vi "GetDAQOutputs.vi"(8 "error in (no error)":errorcluster, 11 "Device.Simulation in":refnum<class "Device.Simulation.lvclass">) -> (0 "error out":errorcluster, 2 "DAQ Outputs":T1, 3 "Device.Simulation out":refnum<class "Device.Simulation.lvclass">)   [LabVIEW 2019, in "Device.Simulation.lvlib" / "Device.Simulation.lvclass"]
uses:
  Device.Simulation.lvclass
  state--cluster.ctl
  Device.Simulation.lvclass/Device.Simulation.ctl
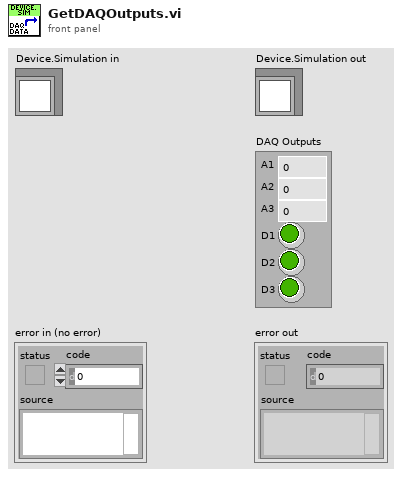
[diagram p1: front panel]
types:
  T1 = typedef "Device.Simulation.lvlib/Device.Simulation.lvclass/state--cluster.ctl" = cluster{"A1":dbl, "A2":dbl, "A3":dbl, "D1":bool, "D2":bool, "D3":bool}
  T2 = typedef "Device.Simulation.lvlib/Device.Simulation.lvclass/privateData--reference.ctl" = refnum<data-value>
  T3 = typedef "Device.Simulation.lvlib/Device.Simulation.lvclass/privateData--cluster.ctl" = cluster{"config":T4, "state":T1}
  T4 = typedef "Device.Simulation.lvlib/Device.Simulation.lvclass/config--cluster.ctl" = cluster{"Name":string, "Time to Connect (ms)":u32, "Time to Check Connection (ms)":u32, "Time to Disconnect (ms)":u32, "Time to Read State (ms)":u32}
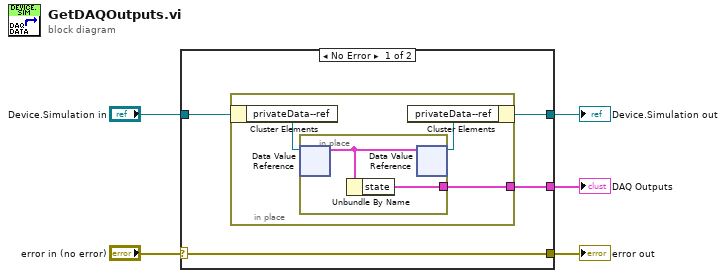
[diagram p0: block diagram]
diagram:
  n1 = case shown="No Error" "error in (no error)" {
    selector: "error in (no error)" -> [w9 w16]
    tunnel: [w9 w16] -> w4
    tunnel: [w7 w15] -> w2
    tunnel: "Device.Simulation in" -> [w8 w15]
    tunnel: [w6 _] -> w1
    frame No Error {
      n2 = in-place {
        in-place-border: [w12] -> w6
        n3 = in-place-cluster #1(w8) -> ("privateData--ref"=w11:T2)
        n4 = in-place {
          in-place-border: [w14] -> w12
          n5 = in-place-dvr #2(w11) -> (w13:T3)  [unwired: 1 out]
          n6 = Unbundle By Name(w13) -> ("state"=w14:T1)
          n7 = in-place-dvr #2(w13) -> (w10:T2)  [unwired: 1 out]
        }
        n8 = in-place-cluster #1("privateData--ref"=w10) -> (w7:refnum<class "Device.Simulation.lvclass">)
      }
    }
    frame Error {
    }
  }
  "error out" <- w4
  "Device.Simulation out" <- w2
  "DAQ Outputs" <- w1
